vi "IC_SetVCDSwitch.vi"(1 "On / Off":bool, 2 "Element ID":u16(ring) items=["Value", "Auto", "One Push", "Whitebalance Bue", "Whitebalance Red", "Auto Reference", "Trigger Polarity", "Trigger Mode", "Reset Value", "GP IO Input", "GP IO Output", "GP IO Write", "GP IO Read", "Strope Polarity", "Strobe Duration", "Strobe Delay"], 3 "Property":u16(ring) items=["Brightness", "Contrast", "Hue", "Saturation", "Sharpness", "Gamma", "Color Enable", "White Balance", "Backlight Compensation", "Gain", "Pan", "Tilt", "Roll", "Zoom", "Exposure", "Iris", "Focus", "Trigger Mode", "VCR Compatibility", "Signal Detected", "Testpattern", "GP IO", "Strobe"], 4 "ICImagingControl3.IICImagingControl":refnum<k7>) -> (0 "ICImagingControl3.IICImagingControl 2":refnum<k7>)   [LabVIEW 2020]
doc: "This VI sets a Switch for the passed VD Property"
uses:
  Instance           2 23Saved   IC_SetVCDSwitch .vi
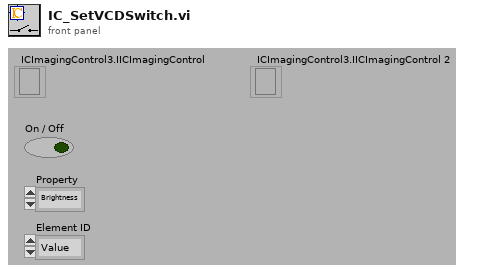
[diagram p1: front panel]
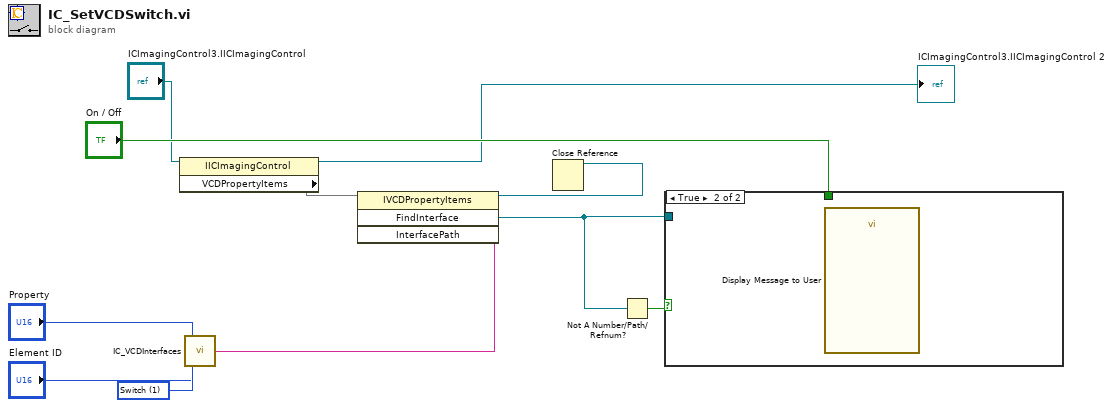
[diagram p0: block diagram]
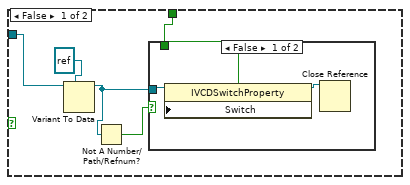
[diagram p2: hidden frame]
diagram:
  w5 = u16 1 items=["Range", "Switch", "Button", "Mapstrings", "Absolute Values"] ("Interface")
  n1 = property class="IICImagingControl"(reference="ICImagingControl3.IICImagingControl") -> (reference out=→"ICImagingControl3.IICImagingControl 2":refnum<k7>, "VCDPropertyItems"=w7)  [unwired: 1 in, 1 out]
  n2 = call "IC_VCDInterfaces.vi"("Interface"=w5, "Element ID"="Element ID", "Property"="Property") -> ("Interface Path"=w6:string)
  n3 = invoke class="IVCDPropertyItems" method="FindInterface"(reference=w7, "InterfacePath"=w6) -> (reference out=w8:refnum<k7>, "FindInterface"=w2:refnum<k7>)  [unwired: 2 in, 2 out]
  n4 = Close Reference(reference=w8) -> ()  [unwired: 1 in, 1 out]
  n5 = Not A Number/Path/Refnum?(number/path/refnum=w2) -> (NaN/Path/Refnum?=w1:bool)
  n6 = case shown="True" w1 {
    tunnel: "On / Off" -> [w12 _]
    tunnel: w2 -> [w13 _]
    frame False {
      n7 = Variant To Data(type=refnum<k7> refnum ("ICImagingControl3.IVCDSwitchProperty"), Variant=w13) -> (data=w15:refnum<k7>)  [unwired: 1 in, 1 out]
      n8 = Not A Number/Path/Refnum?(number/path/refnum=w15) -> (NaN/Path/Refnum?=w16:bool)
      n9 = case shown="False" w16 {
        tunnel: w15 -> [w18 _]
        tunnel: w12 -> [w17 _]
        frame False {
          n10 = property class="IVCDSwitchProperty"(reference=w18, "Switch"=w17) -> (reference out=w19:refnum<k7>)  [unwired: 1 in, 1 out]
          n11 = Close Reference(reference=w19) -> ()  [unwired: 1 in, 1 out]
        }
        frame True {
        }
      }
    }
    frame True {
      n12 = call "Display Message to User"() -> ()  [unwired: 10 in, 2 out]
    }
  }
